vi "Read Group Index.vi"(8 "error in (no error)":errorcluster, 11 "bt_Blackboard_Leaf Type in":refnum<class "bt_Blackboard_Leaf Type.lvclass">) -> (0 "error out":errorcluster, 2 "Group Index":i32, 3 "bt_Blackboard_Leaf Type out":refnum<class "bt_Blackboard_Leaf Type.lvclass">)   [LabVIEW 2021, in "BT.lvlib" / "bt_Blackboard_Leaf Type.lvclass"]
uses:
  bt_Blackboard_Leaf Type.lvclass
  bt_Blackboard_Leaf Type.lvclass/bt_Blackboard_Leaf Type.ctl
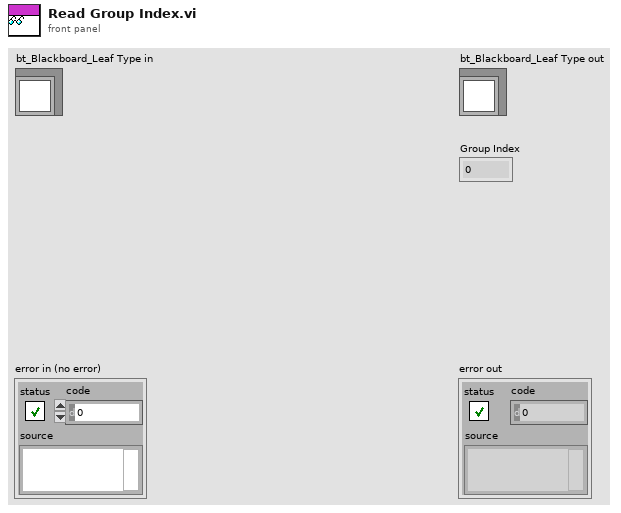
[diagram p1: front panel]
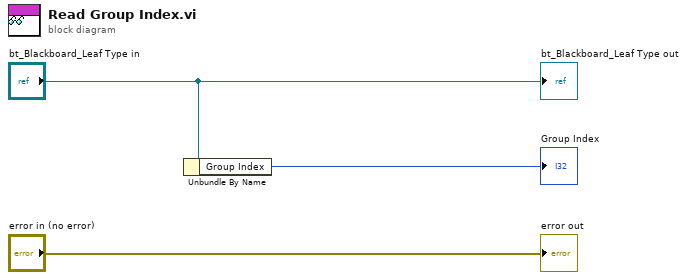
[diagram p0: block diagram]
diagram:
  n1 = Unbundle By Name("bt_Blackboard_Leaf Type in") -> ("Group Index"=→"Group Index":i32)
  "error out" <- "error in (no error)"
  "bt_Blackboard_Leaf Type out" <- "bt_Blackboard_Leaf Type in"
